vi "Dialog-UserChooseMeter#.vi"(8 "error in (no error)":errorcluster, 11 "Meter-Test in":refnum<class "Meter-Test.lvclass">) -> (0 "error out":errorcluster, 3 "Meter-Test out":refnum<class "Meter-Test.lvclass">)   [LabVIEW 2013, in "Meter-Test.lvclass"]
uses:
  Meter-Test.lvclass
  Meter-Test.lvclass/Meter-Test.ctl
panel:
  in  "Finished Button":bool
  in  "Number of Meters Installed":i32=1 min=1 max=8
  # "Please indicate how many meters are installed in the EGM"
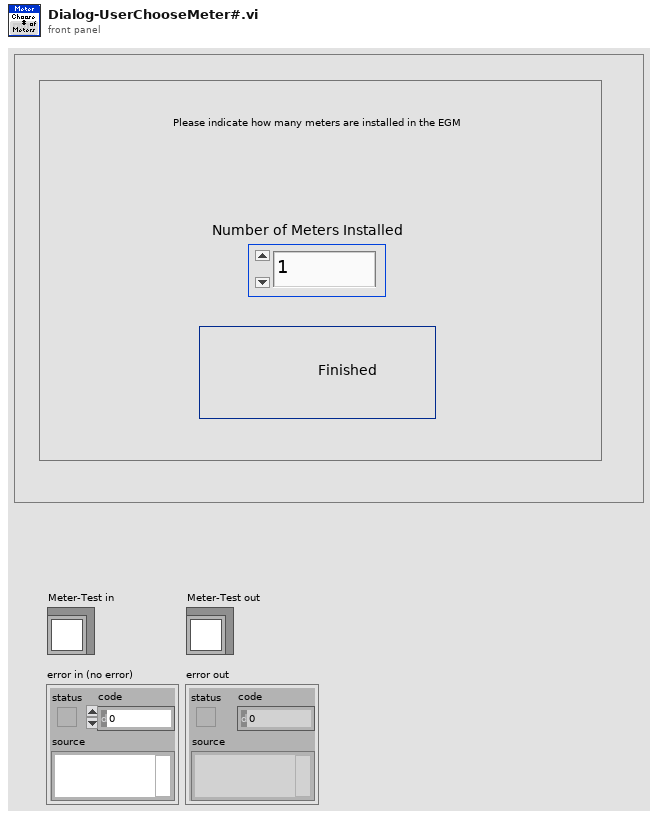
[diagram p1: front panel]
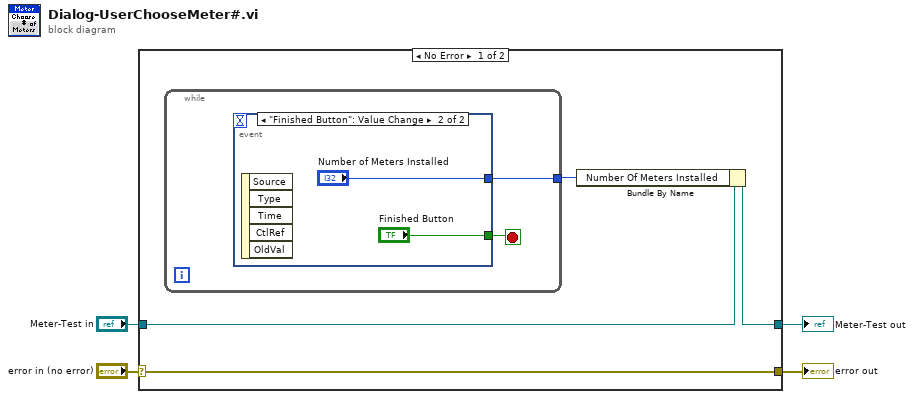
[diagram p0: block diagram]
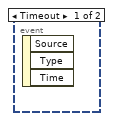
[diagram p2: hidden frame]
diagram:
  n1 = case shown="No Error" "error in (no error)" {
    selector: "error in (no error)" -> [w8 w14]
    tunnel: [w8 w14] -> w3
    tunnel: [w5 w13] -> w1
    tunnel: "Meter-Test in" -> [w7 w13]
    frame No Error {
      n2 = while {
        tunnel: [w9] -> w6
        stop <- w10 stop-if-true
        n3 = event shown="[1] \"Finished Button\": Value Change" {
          selector: _ -> [_ _]
          dyn-events: _ -> [_ _]
          timeout: _ -> [_ _]
          tunnel: [_ "Finished Button"] -> w10
          tunnel: [_ "Number of Meters Installed"] -> w9
          event Timeout {
            n4 = event-data() -> ()  [unwired: 1 in, 3 out]
          }
          event "Finished Button": Value Change {
            n5 = event-data() -> ()  [unwired: 1 in, 5 out]
          }
        }
      }
      n6 = Bundle By Name(cluster=w7, "Number Of Meters Installed"=w6) -> (w5:refnum<class "Meter-Test.lvclass">)
    }
    frame Error {
    }
  }
  "error out" <- w3
  "Meter-Test out" <- w1
